vi "Process-received-message.vi"(7 "Data ref in":T1, 8 "error in (no error)":errorcluster, 10 "Message":refnum<class "Message.lvclass">, 11 "Client in":T2) -> (0 "error out":errorcluster, 3 "Client out":T2, 5 "Data ref out":T1)   [LabVIEW 2013, in "SLMControl.lvlib" / "SC-Main.lvclass"]
doc: "This function wraps the message checks, analysis and response action functions.\nThe validity of the message and message origin is checked, after which the appropriate module action is determined and executed.\n\nThe actions should be implemented by the module integrator."
uses:
  SC-Main.lvclass
  Client/Sources/Object-reference.ctl
  Client/Sources/SC-Client.lvclass
  SA-SLMAPI/Sources/Message.lvclass
  Object-reference.ctl
  SC-Main.lvclass/SC-Main.ctl
  SA-SLMAPI/Sources/Send-status/Send-status.lvclass
  SA-SLMAPI/Sources/Send-status/Send-status.lvclass/Send-status.ctl
  Main-actions.ctl
  Enqueue-modes.ctl
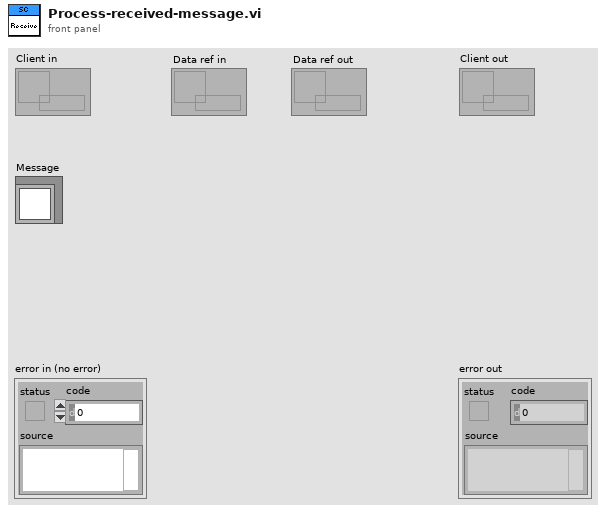
[diagram p1: front panel]
types:
  T1 = typedef "SLMControl.lvlib/SC-Main.lvclass/Object-reference.ctl" = refnum<data-value>
  T2 = typedef "SLMControl.lvlib/SC-Client.lvclass/Object-reference.ctl" = refnum<data-value>
  T3 = typedef "SLMControl.lvlib/SC-Main.lvclass/Enqueue-modes.ctl" = enum16{"Default", "Priority", "Flush"}
  T4 = typedef "SLMControl.lvlib/SC-Client.lvclass/Supported-messages.ctl" = enum16{"Heartbeat", "Error", "Start client", "Client stopped", "Action", "Query status", "Send status", "Get clients"}
  T5 = typedef "SLMControl.lvlib/SC-Client.lvclass/Supported-modules.ctl" = enum16{"Server", "All", "SLMControl", "PowderDeposition", "StrategyParser", "CameraVision", "MaterialCharacterization", "StatusMonitor", "SLMSimulation", "LaserCharacterization"}
  T6 = typedef "PowderDeposition.lvlib/PD-Data.lvclass/Statusses.ctl" = enum16{"Idle", "Initialized", "Configured", "Activated", "Started", "Paused", "Stopped", "Reset", "Error", "Exited"}
  T7 = typedef "SLMControl.lvlib/SC-Client.lvclass/Supported-actions.ctl" = enum16{"Idle", "Initialize", "Load settings", "Load file", "Activate", "Start", "Pause", "Stop", "Repeat", "Reset", "Exit"}
  T8 = typedef "SLMControl.lvlib/SC-Main.lvclass/Main-actions.ctl" = enum16{"Idle", "Initialize", "Load configuration", "Save configuration", "Load lasing files", "Load deposition files", "Refresh files", "Clear files", "Open lasing file", "Activate", "Start", "Start deposition cycle", "Start lasing cycle", "Iterate", "Abort", "Stop", "Exit"}
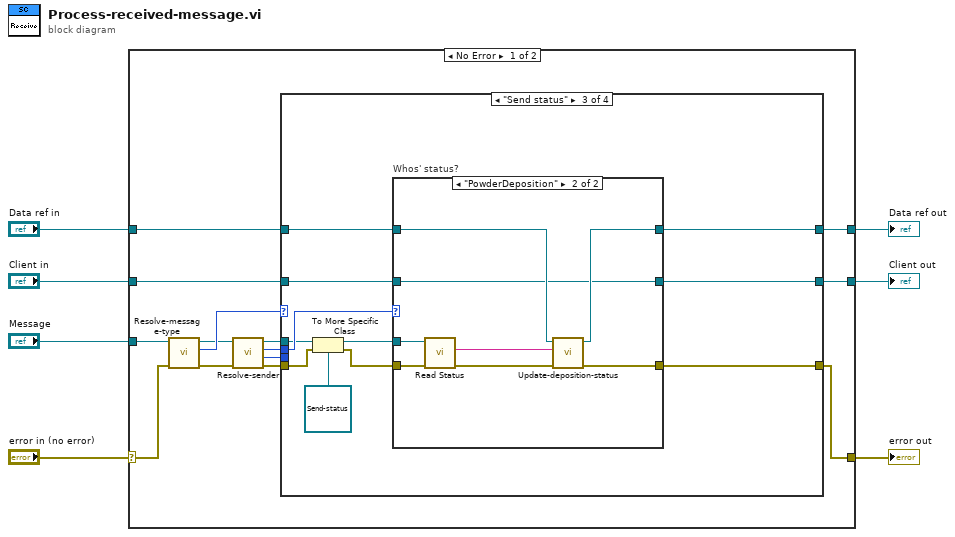
[diagram p0: block diagram]
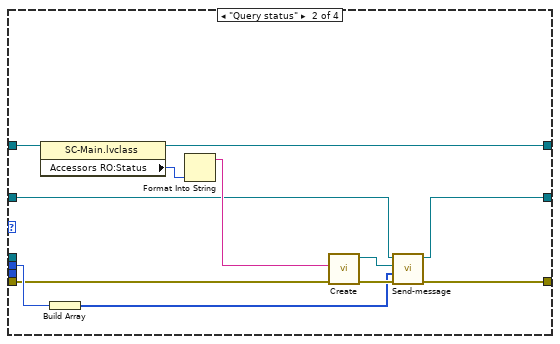
[diagram p3: hidden frame]
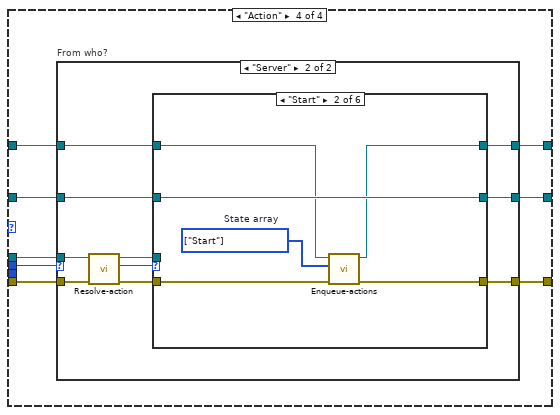
[diagram p5: hidden frame]
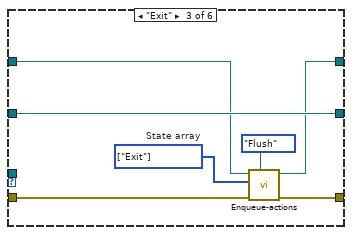
[diagram p8: hidden frame]
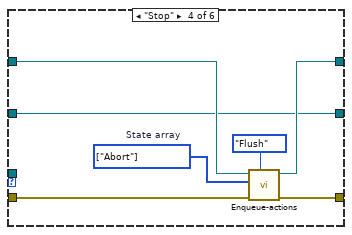
[diagram p9: hidden frame]
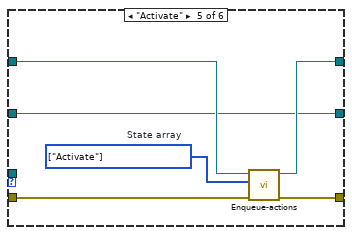
[diagram p10: hidden frame]
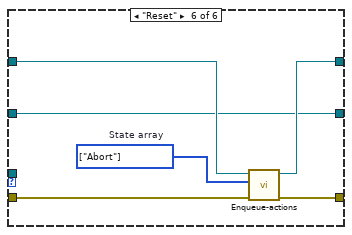
[diagram p11: hidden frame]
diagram:
  n1 = case shown="No Error" "error in (no error)" {
    selector: "error in (no error)" -> [w19 w117]
    tunnel: [w8 w117] -> w6
    tunnel: [w20 w116] -> w4
    tunnel: "Client in" -> [w21 w116]
    tunnel: "Message" -> [w18 _]
    tunnel: "Data ref in" -> [w10 w115]
    tunnel: [w9 w115] -> w1
    frame No Error {
      n2 = call "Resolve-message-type.vi"("error in (no error)"=w19, "Message"=w18) -> ("error out"=w15:errorcluster, "Message type"=w17:T4, "Message dup"=w16:refnum<class "Message.lvclass">)  [unwired: 7 in]
      n3 = call "Resolve-sender.vi"("error in (no error)"=w15, "Message"=w16) -> ("error out"=w12:errorcluster, "Sender ID"=w13:i32, "Sender type"=w14:T5, "Message dup"=w11:refnum<class "Message.lvclass">)  [unwired: 6 in]
      n4 = case shown="\"Send status\"" w17 {
        tunnel: [w23 w28 w43 w60] -> w8
        tunnel: w21 -> [w24 w31 w45 w65]
        tunnel: [w24 w30 w44 w63] -> w20
        tunnel: w14 -> [_ w27 w42 w59]
        tunnel: w13 -> [_ _ _ _]
        tunnel: w12 -> [w23 w26 w38 w62]
        tunnel: w11 -> [_ _ w41 w61]
        tunnel: w10 -> [w22 w36 w47 w66]
        tunnel: [w22 w35 w46 w64] -> w9
        frame Default {
        }
        frame "Query status" {
          n5 = property class="SC-Main.lvclass"(reference=w36) -> (reference out=w35:T1, "Accessors RO:Status"=w34:T6)  [unwired: 1 in, 1 out]
          n6 = Build Array(w27) -> (w25:T5[])
          n7 = Format Into String(w34) -> (resulting string=w33:string)  [unwired: 3 in, 1 out]
          n8 = call "Create.vi"("error in (no error)"=w26, "Status"=w33) -> ("error out"=w32:errorcluster, "Send-status out"=w29:refnum<class "Send-status.lvclass">)  [unwired: 8 in]
          n9 = call "Send-message.vi"("error in (no error)"=w32, "Receivers"=w25, "Message"=w29, "Client in"=w31) -> ("error out"=w28:errorcluster, "Client out"=w30:T2)  [unwired: 6 in]
        }
        frame "Send status" {
          n10 = To More Specific Class(target class=refnum<class "Send-status.lvclass"> refnum ("Messages.lvlib:Send-status.lvclass"), reference=w41, error in=w38) -> (specific class reference=w40:refnum<class "Send-status.lvclass">, error out=w37:errorcluster)
          n11 = case "Whos' status?" shown="\"PowderDeposition\"" w42 {
            tunnel: w47 -> [w50 w58]
            tunnel: w40 -> [_ w57]
            tunnel: w37 -> [w48 w56]
            tunnel: [w50 w54] -> w46
            tunnel: w45 -> [w49 w53]
            tunnel: [w49 w53] -> w44
            tunnel: [w48 w52] -> w43
            frame Default {
            }
            frame "PowderDeposition" {
              n12 = call "Read Status.vi"("error in (no error)"=w56, "Send-status in"=w57) -> ("error out"=w55:errorcluster, "Status"=w51:string)  [unwired: 7 in, 1 out]
              n13 = call "Update-deposition-status.vi"("error in (no error)"=w55, "Status"=w51, "Data in"=w58) -> ("error out"=w52:errorcluster, "Data out"=w54:T1)  [unwired: 7 in]
            }
          }
        }
        frame "Action" {
          n14 = case "From who?" shown="\"Server\"" w59 {
            tunnel: w66 -> [w69 w79]
            tunnel: w65 -> [w68 w78]
            tunnel: [w69 w77] -> w64
            tunnel: [w68 w76] -> w63
            tunnel: w62 -> [w67 w72]
            tunnel: w61 -> [_ w71]
            tunnel: [w67 w70] -> w60
            frame Default {
            }
            frame "Server" {
              n15 = call "Resolve-action.vi"("error in (no error)"=w72, "Message"=w71) -> ("error out"=w73:errorcluster, "Action"=w74:T7, "Message dup"=w75:refnum<class "Message.lvclass">)  [unwired: 7 in]
              n16 = case shown="\"Start\"" w74 {
                tunnel: w79 -> [w82 w85 w90 w99 w106 w112]
                tunnel: w78 -> [w81 w88 w95 w97 w104 w110]
                tunnel: [w82 w86 w91 w98 w105 w111] -> w77
                tunnel: [w81 w88 w95 w97 w104 w110] -> w76
                tunnel: w75 -> [_ _ _ _ _ _]
                tunnel: w73 -> [w80 w84 w89 w96 w103 w109]
                tunnel: [w80 w83 w92 w100 w107 w113] -> w70
                frame Default {
                }
                frame "Start" {
                  w87 = T8[] [enum."Start"] items=["Idle", "Initialize", "Load configuration", "Save configuration", "Load lasing files", "Load deposition files", "Refresh files", "Clear files", "Open lasing file", "Activate", "Start", "Start deposition cycle", "Start lasing cycle", "Iterate", "Abort", "Stop", "Exit"]  # State array
                  n17 = call "Enqueue-actions.vi"("error in (no error)"=w84, "State array"=w87, "State queue in"=w85) -> ("error out"=w83:errorcluster, "State queue out"=w86:T1)  [unwired: 6 in, 1 out]
                }
                frame "Exit" {
                  w94 = T8[] [enum."Exit"] items=["Idle", "Initialize", "Load configuration", "Save configuration", "Load lasing files", "Load deposition files", "Refresh files", "Clear files", "Open lasing file", "Activate", "Start", "Start deposition cycle", "Start lasing cycle", "Iterate", "Abort", "Stop", "Exit"]  # State array
                  n18 = call "Enqueue-actions.vi"("Enqueue mode"=Enqueue-modes."Flush", "error in (no error)"=w89, "State array"=w94, "State queue in"=w90) -> ("error out"=w92:errorcluster, "State queue out"=w91:T1)  [unwired: 5 in, 1 out]
                }
                frame "Stop" {
                  w102 = T8[] [enum."Abort"] items=["Idle", "Initialize", "Load configuration", "Save configuration", "Load lasing files", "Load deposition files", "Refresh files", "Clear files", "Open lasing file", "Activate", "Start", "Start deposition cycle", "Start lasing cycle", "Iterate", "Abort", "Stop", "Exit"]  # State array
                  n19 = call "Enqueue-actions.vi"("Enqueue mode"=Enqueue-modes."Flush", "error in (no error)"=w96, "State array"=w102, "State queue in"=w99) -> ("error out"=w100:errorcluster, "State queue out"=w98:T1)  [unwired: 5 in, 1 out]
                }
                frame "Activate" {
                  w108 = T8[] [enum."Activate"] items=["Idle", "Initialize", "Load configuration", "Save configuration", "Load lasing files", "Load deposition files", "Refresh files", "Clear files", "Open lasing file", "Activate", "Start", "Start deposition cycle", "Start lasing cycle", "Iterate", "Abort", "Stop", "Exit"]  # State array
                  n20 = call "Enqueue-actions.vi"("error in (no error)"=w103, "State array"=w108, "State queue in"=w106) -> ("error out"=w107:errorcluster, "State queue out"=w105:T1)  [unwired: 6 in, 1 out]
                }
                frame "Reset" {
                  w114 = T8[] [enum."Abort"] items=["Idle", "Initialize", "Load configuration", "Save configuration", "Load lasing files", "Load deposition files", "Refresh files", "Clear files", "Open lasing file", "Activate", "Start", "Start deposition cycle", "Start lasing cycle", "Iterate", "Abort", "Stop", "Exit"]  # State array
                  n21 = call "Enqueue-actions.vi"("error in (no error)"=w109, "State array"=w114, "State queue in"=w112) -> ("error out"=w113:errorcluster, "State queue out"=w111:T1)  [unwired: 6 in, 1 out]
                }
              }
            }
          }
        }
      }
    }
    frame Error {
    }
  }
  "error out" <- w6
  "Client out" <- w4
  "Data ref out" <- w1
